vi "Is Synced to Scan.vi"(8 "error in":errorcluster, 11 "Item Ref in":T1 format="%.0x") -> (0 "error out":errorcluster, 1 "Engine Rate":dbl, 2 "Sync to Scan?":bool, 3 "Item Ref out":T1 format="%.0x")   [LabVIEW 2019, in "Scan Engine Custom Device.lvlib"]
uses:
  Scan Engine Custom Device.lvlib
  <vilib>/NI VeriStand/Custom Device API/Custom Device Item Ref.ctl
  NationalInstruments.VeriStand.SystemDefinitionAPI
  NationalInstruments.VeriStand.SystemStorage
  <vilib>/NI VeriStand/Custom Device Tools/Custom Device Utility Library/Custom Device Utility Library.lvlib
  <vilib>/NI VeriStand/Custom Device API/Custom Device API.lvlib
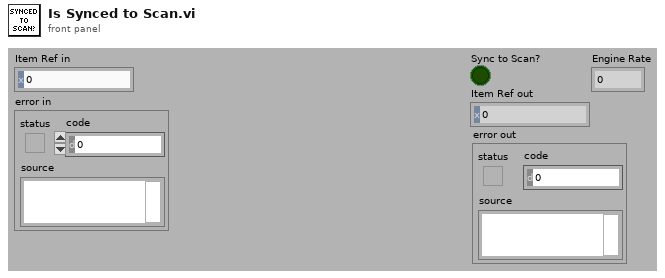
[diagram p1: front panel]
types:
  T1 = typedef "Custom Device API.lvlib/Custom Device Item Ref.ctl" = u64
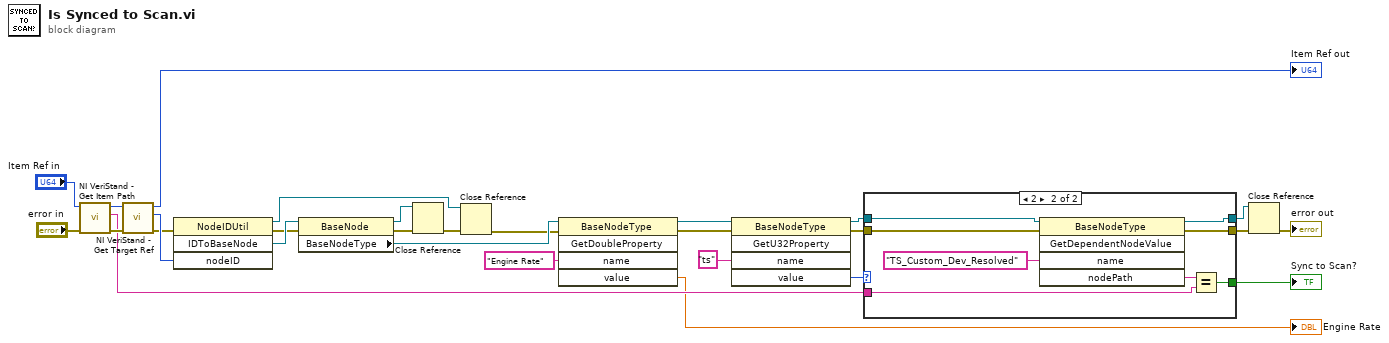
[diagram p0: block diagram]
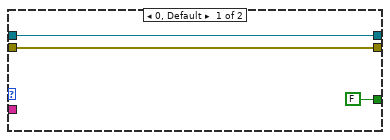
[diagram p2: hidden frame]
diagram:
  n1 = call <vilib>:"NI VeriStand - Get Item Path.vi"("error in (no error)"="error in", "Item Ref in"="Item Ref in") -> ("error out"=w21:errorcluster, "Path"=w18:string, "Item Ref out"=w22:T1)  [unwired: 6 in, 1 out]
  n2 = call <vilib>:"NI VeriStand - Get Target Ref.vi"("error in"=w21, "Item Ref in"=w22) -> ("error out"=w8:errorcluster, "Target Ref"=w9:T1, "Item Ref out"=→"Item Ref out":T1)  [unwired: 6 in, 1 out]
  n3 = invoke class="NodeIDUtil" method="IDToBaseNode"(error in=w8, "nodeID"=w9) -> (reference out=w6:refnum<k24>, error out=w10:errorcluster, "IDToBaseNode"=w11:refnum<k24>)  [unwired: 2 in, 1 out]
  n4 = property class="BaseNode"(reference=w11, error in=w10) -> (reference out=w4:refnum<k24>, error out=w5:errorcluster, "BaseNodeType"=w7:refnum<k24>)
  n5 = Close Reference(reference=w4, error in (no error)=w5) -> (error out=w3:errorcluster)
  n6 = Close Reference(reference=w6, error in (no error)=w3) -> (error out=w2:errorcluster)
  n7 = invoke class="BaseNodeType" method="GetDoubleProperty"(reference=w7, error in=w2, "name"="Engine Rate") -> (reference out=w14:refnum<k24>, error out=w15:errorcluster, "value"=→"Engine Rate":dbl)  [unwired: 2 in, 2 out]
  n8 = invoke class="BaseNodeType" method="GetU32Property"(reference=w14, error in=w15, "name"="ts") -> (reference out=w28:refnum<k24>, error out=w27:errorcluster, "value"=w25:u32)  [unwired: 2 in, 2 out]
  n9 = case shown="2" w25 {
    tunnel: w28 -> [w30 w39]
    tunnel: w27 -> [w29 w38]
    tunnel: [FALSE w34] -> w24
    tunnel: w18 -> [_ w35]
    tunnel: [w30 w33] -> w17
    tunnel: [w29 w32] -> w16
    frame 0, Default {
    }
    frame 2 {
      n10 = invoke class="BaseNodeType" method="GetDependentNodeValue"(reference=w39, error in=w38, "name"="TS_Custom_Dev_Resolved") -> (reference out=w33:refnum<k24>, error out=w32:errorcluster, "nodePath"=w36:string)  [unwired: 2 in, 2 out]
      n11 = Equal?(x=w36, y=w35) -> (x = y?=w34:bool)
    }
  }
  "Sync to Scan?" <- w24
  n12 = Close Reference(reference=w17, error in (no error)=w16) -> (error out=→"error out":errorcluster)
